vi "Release.vi"(8 "error in (no error)":errorcluster, 11 "MotionSystem in":refnum<class "MotionSystem.lvclass">) -> (0 "error out":errorcluster, 3 "MotionSystem out":refnum<class "MotionSystem.lvclass">)   [LabVIEW 2016, in "MotionSystem.lvlib" / "MotionSystem.lvclass"]
uses:
  <userlib>/Common Components/Hardware/Abstract System/MotionSystem/MotionSystem/MotionSystem.lvclass
  <userlib>/Common Components/Hardware/Abstract System/MotionSystem/MotionSystem/MotionSystem.lvclass/MotionSystem.ctl
  <userlib>/Common Components/Hardware/Motor/Motor/Motor.lvclass
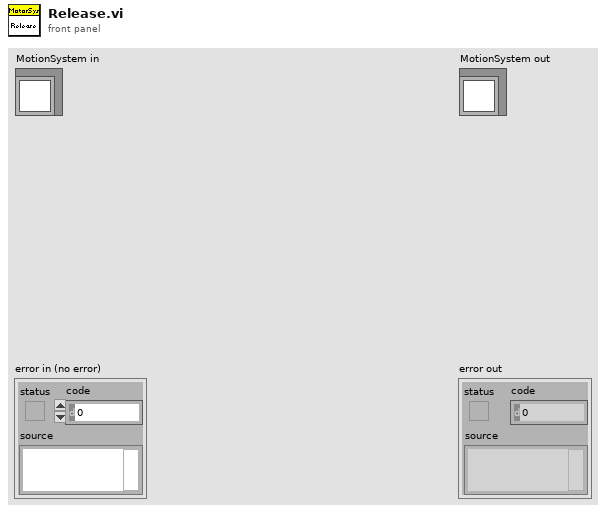
[diagram p1: front panel]
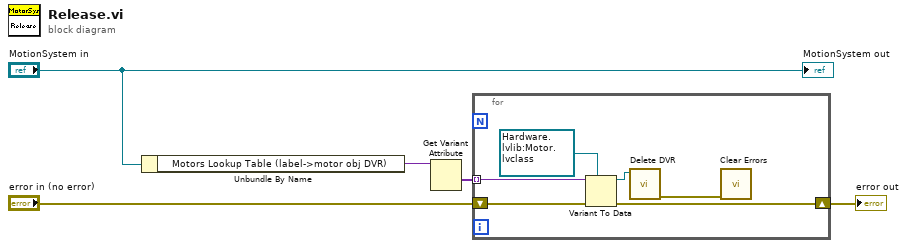
[diagram p0: block diagram]
diagram:
  n1 = Unbundle By Name("MotionSystem in") -> ("Motors Lookup Table (label->motor obj DVR)"=w4:variant)
  n2 = Get Variant Attribute(Variant=w4) -> (values=w3:variant[])  [unwired: 3 in, 3 out]
  n3 = for {
    tunnel: w3 -> [w11] mode=indexing
    shift-right: [w9] -> w1
    shift-left: "error in (no error)" -> [w10]
    n4 = Variant To Data(error in=w10, type=refnum<data-value> refnum ("data value reference"), Variant=w11) -> (data=w7:refnum<data-value>, error out=w9:errorcluster)
    n5 = call <userlib>:"Delete DVR.vi"("data value reference"=w7) -> ("error out"=w6:errorcluster)  [unwired: 9 in, 1 out]
    n6 = call <vilib>:"Clear Errors.vi"("error in (no error)"=w6) -> ()  [unwired: 5 in, 2 out]
  }
  "error out" <- w1
  "MotionSystem out" <- "MotionSystem in"
